vi "Read Arguments.vi"(8 "error in (no error)":errorcluster, 11 "CLI in":refnum<class "CLI.lvclass">) -> (0 "error out":errorcluster, 2 "Arguments":string[](array[string]), 3 "CLI out":refnum<class "CLI.lvclass">)   [LabVIEW 2011, in "CLI.lvclass"]
uses:
  CLI.lvclass
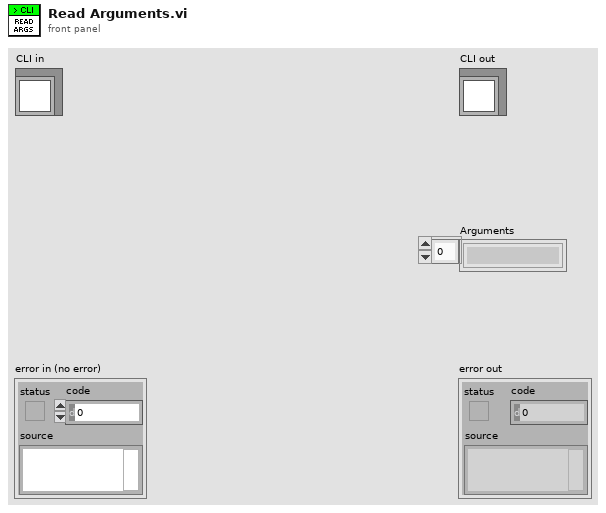
[diagram p1: front panel]
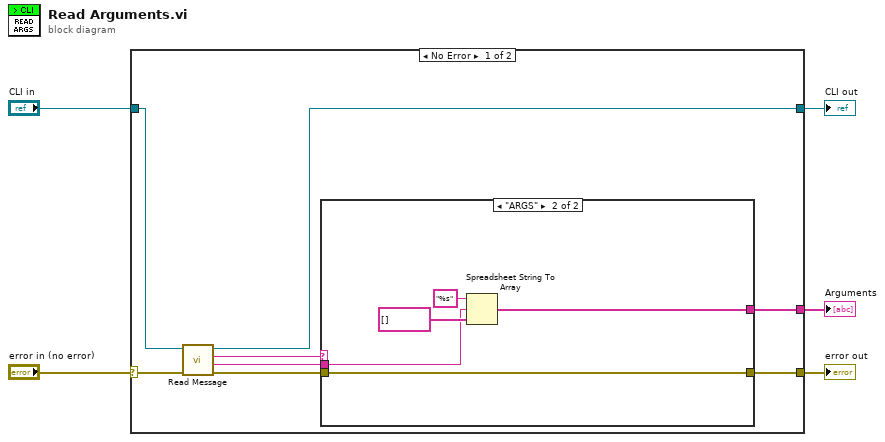
[diagram p0: block diagram]
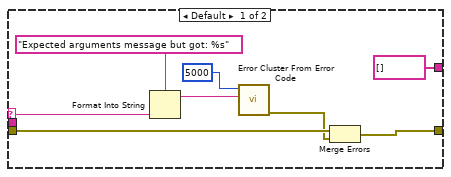
[diagram p2: hidden frame]
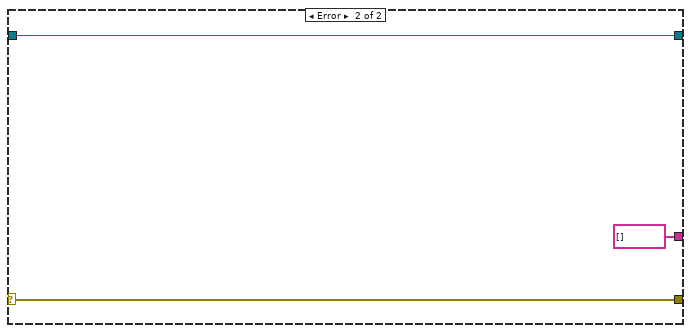
[diagram p3: hidden frame]
diagram:
  n1 = case shown="No Error" "error in (no error)" {
    selector: "error in (no error)" -> [w13 w29]
    tunnel: [w9 w29] -> w4
    tunnel: [w11 w28] -> w2
    tunnel: "CLI in" -> [w12 w28]
    tunnel: [w7 string[] []] -> w1
    frame No Error {
      n2 = call "Read Message.vi"("error in (no error)"=w13, "CLI in"=w12) -> ("error out"=w8:errorcluster, "Message Contents"=w6:string, "Message Type"=w10:string, "CLI out"=w11:refnum<class "CLI.lvclass">)  [unwired: 6 in]
      n3 = case shown="\"ARGS\"" w10 {
        selector: w10 -> [w17 _]
        tunnel: [w16 w26] -> w9
        tunnel: w8 -> [w21 w26]
        tunnel: [string[] [] w23] -> w7
        tunnel: w6 -> [_ w22]
        frame Default {
          n4 = Format Into String(format string="Expected arguments message but got: %s", w17) -> (resulting string=w18:string)  [unwired: 2 in, 1 out]
          n5 = call <vilib>:"Error Cluster From Error Code.vi"("error message (\"\")"=w18, "error code (0)"=5000) -> ("error out"=w15:errorcluster)  [unwired: 7 in]
          n6 = Merge Errors(w21, w15) -> (w16:errorcluster)
        }
        frame "ARGS" {
          n7 = Spreadsheet String To Array(format string="%s", spreadsheet string=w22, array type (2D Dbl)=string[] []) -> (array=w23:string[])  [unwired: 1 in]
        }
      }
    }
    frame Error {
    }
  }
  "error out" <- w4
  "CLI out" <- w2
  "Arguments" <- w1
